vi "Convert MAC Address.vi"(11 "DUT MAC ADDRESS":string="02:00:08:38:2d:37") -> (3 "destination MAC address":cluster{u8, u8, u8, u8, u8, u8} {"?" format="%x"; "?" format="%x"; "?" format="%x"; "?" format="%x"; "?" format="%x"; "?" format="%x"})   [LabVIEW 2026]
panel:
  out "Array":u8[](array[numeric]) format="%x"
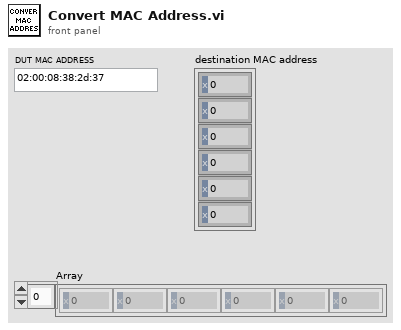
[diagram p1: front panel]
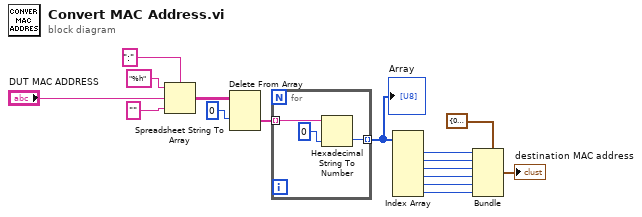
[diagram p0: block diagram]
diagram:
  n1 = Spreadsheet String To Array(delimiter (Tab)=":", format string="%h", spreadsheet string="DUT MAC ADDRESS", array type (2D Dbl)="" ("delimiter (Tab)")) -> (array=w12:string[][])
  n2 = Delete From Array(array=w12, index (row)=0 ("disabled index (col)")) -> (deleted portion=w10:string[])  [unwired: 2 in, 1 out]
  n3 = for {
    tunnel: w10 -> [w19] mode=indexing
    tunnel: [w18] -> w1 mode=indexing
    n4 = Hexadecimal String To Number(string=w19, default (0uL)=u8 0 ("default (0 U32)")) -> (number=w18:u8)  [unwired: 1 in, 1 out]
  }
  "Array" <- w1
  n5 = Index Array(array=w1) -> (element #1=w8:u8, element #2=w7:u8, element #3=w6:u8, element #4=w5:u8, element #5=w4:u8, element #6=w3:u8)  [unwired: 6 in]
  n6 = Bundle(cluster=cluster{u8, u8, u8, u8, u8, u8} {0, 0, 0, 0, 0, 0} ("destination MAC address"), w8, w7, w6, w5, w4, w3) -> (→"destination MAC address":cluster{u8, u8, u8, u8, u8, u8})
